vi "Dispatcher Read and Process UDP Messages.vi"(0 "UDP conn ID":refnum<k16>, 9 "timeout (10 ms)":i32=10, 11 "error in":errorcluster) -> (4 "message string":string, 6 "message":T1, 15 "error out":errorcluster)   [LabVIEW 2009, in "AMC.lvlib"]
uses:
  AMC.lvlib
  Message.ctl
  <vilib>/NI/Tools/Keyed Array/KeyedArray.ctl
  <vilib>/NI/Tools/Keyed Array/Tools_KeyedArray.lvlib
panel:
  out "message length":i32
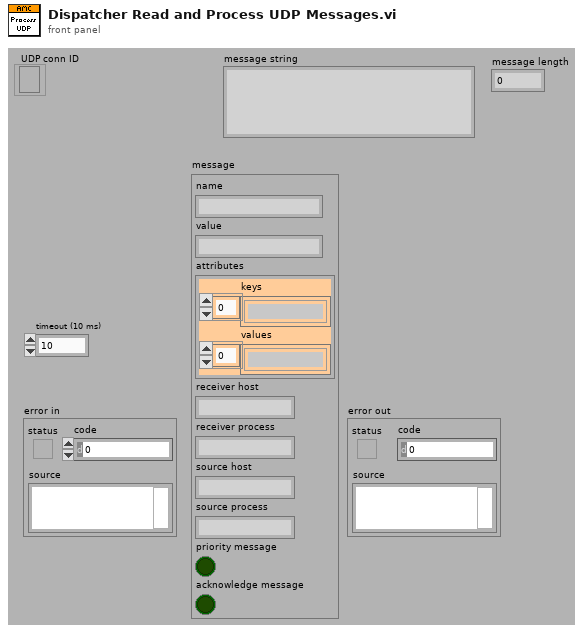
[diagram p1: front panel]
types:
  T1 = typedef "AMC.lvlib/Message.ctl" = cluster{"name":string, "value":string, "attributes":T2, "receiver host":string, "receiver process":string, "source host":string, "source process":string, "priority message":bool, "acknowledge message":bool}
  T2 = typedef "Tools_KeyedArray.lvlib/KeyedArray.ctl" = cluster{"keys":string[], "values":string[]}
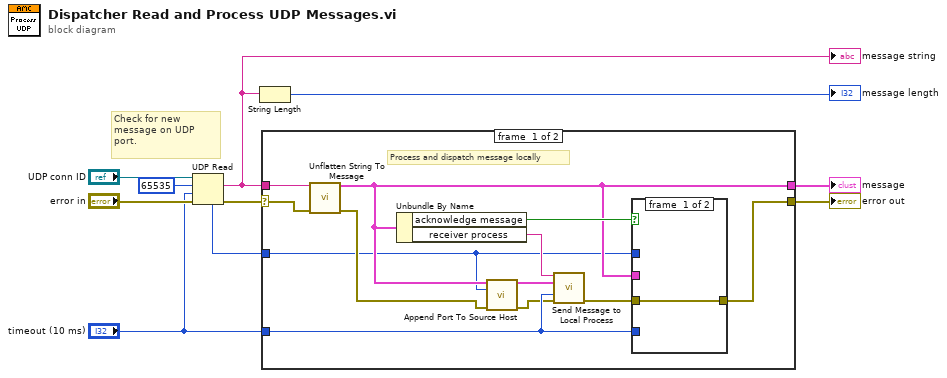
[diagram p0: block diagram]
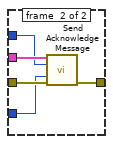
[diagram p2: hidden frame]
diagram:
  # "Check for new message on UDP port."
  n1 = UDP Read(connection ID="UDP conn ID", max size (548)=65535, timeout ms (25000)="timeout (10 ms)", 8:"error in") -> (data out=w3:string, error out=w9:errorcluster, 4:w1:u16)  [unwired: 2 out]
  "message string" <- w3
  n2 = String Length(string=w3) -> (length=→"message length":i32)
  n3 = case shown="No Error" w9 {
    selector: w9 -> [w21 w29]
    tunnel: w3 -> [w22 _]
    tunnel: [w18 w29] -> w7
    tunnel: [w15 _] -> w5
    tunnel: "timeout (10 ms)" -> [w16 _]
    tunnel: w1 -> [w11 _]
    frame #0 {
      # "Process and dispatch message locally"
      n4 = call "Unflatten String To Message.vi"("message string"=w22, "error in"=w21) -> ("message"=w15:T1, "error out"=w13:errorcluster)  [unwired: 12 in]
      n5 = Unbundle By Name(w15) -> ("acknowledge message"=w17:bool, "receiver process"=w20:string)
      n6 = call "Append Port To Source Host.vi"("message in"=w15, "source port"=w11, "error in"=w13) -> ("message out"=w14:T1, "error out"=w12:errorcluster)  [unwired: 11 in]
      n7 = call "Send Message to Local Process.vi"("process name"=w20, "message"=w14, "timeout (-1 ms)"=w16, "error in"=w12) -> ("error out"=w19:errorcluster)  [unwired: 10 in, 1 out]
      n8 = case shown="True" w17 {
        tunnel: w19 -> [w23 w28]
        tunnel: [w23 w27] -> w18
        tunnel: w15 -> [_ w26]
        tunnel: w11 -> [_ w25]
        tunnel: w16 -> [_ w24]
        frame #0 {
        }
        frame #1 {
          n9 = call "Send Acknowledge Message.vi"("received message"=w26, "receiver port"=w25, "timeout"=w24, "error in"=w28) -> ("error out"=w27:errorcluster)  [unwired: 10 in, 1 out]
        }
      }
    }
    frame #1 {
    }
  }
  "error out" <- w7
  "message" <- w5
